vi "macro_PIDController_Execute.vi"   [LabVIEW 2019, in "Trajectory_Library.lvlib"]
uses:
  Trajectory_Library.lvlib
types:
  T1 = typedef "Trajectory_Library.lvlib/PID_TUNING.ctl" = cluster{"Kp":dbl, "Ki":dbl, "Kd":dbl, "MaximumIntegral":dbl, "MinimumIntegral":dbl}
  T2 = typedef "Trajectory_Library.lvlib/PID_INPUT_LIMITS.ctl" = cluster{"MaxInput":dbl, "MinInput":dbl, "Continuous":bool}
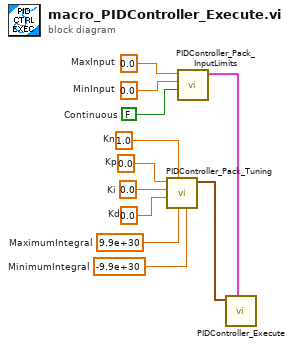
[diagram p0: block diagram]
diagram:
  w1 = 1.0  # Kn
  w2 = 0.0  # MaxInput
  w3 = 0.0  # MinInput
  w4 = FALSE  # Continuous
  w5 = 0.0  # Kp
  w6 = 0.0  # Ki
  w7 = 0.0  # Kd
  w8 = 9.9e+30  # MaximumIntegral
  w9 = -9.9e+30  # MinimumIntegral
  n1 = call "PIDController_Pack_Tuning.vi"("MinimumIntegral"=w9, "MaximumIntegral"=w8, "Kn"=w1, "Kd"=w7, "Ki"=w6, "Kp"=w5) -> ("PID Tuning"=w10:T1)  [unwired: 5 in]
  n2 = call "PIDController_Pack_InputLimits.vi"("Continuous"=w4, "MinInput"=w3, "MaxInput"=w2) -> ("PID Input Limits"=w11:T2)  [unwired: 8 in]
  n3 = call "PIDController_Execute.vi"("PID Input Limits"=w11, "PID Tuning"=w10) -> ()  [unwired: 7 in, 3 out]
